vi "SaveRawData.vi"(4 "error in (no error)":errorcluster, 6 "raw data to be saved":T1[](array[typedef]), 7 "path in":path) -> (0 "error out":errorcluster, 3 "path out":path)   [LabVIEW 2020, in "Initialization.lvlib" / "FileManagement.lvlib"]
uses:
  FileManagement.lvlib
  SignalConversion/DAQChannelRawData.ctl
  SignalConversion/SignalConverson.lvlib
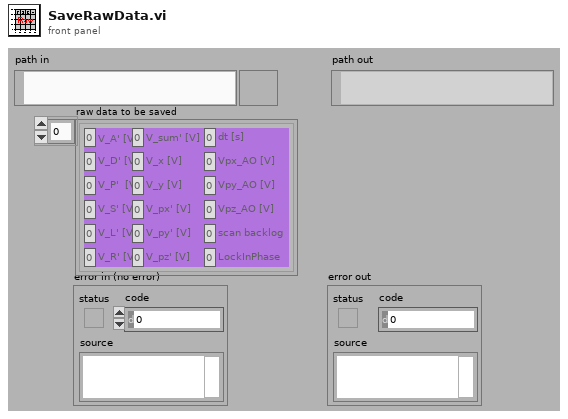
[diagram p1: front panel]
types:
  T1 = typedef "SignalConverson.lvlib/DAQChannelRawData.ctl" = cluster{"V_A' [V]":dbl, "V_D' [V]":dbl, "V_P'  [V]":dbl, "V_S' [V]":dbl, "V_L' [V]":dbl, "V_R' [V]":dbl, "V_sum' [V]":dbl, "V_x [V]":dbl, "V_y [V]":dbl, "V_px' [V]":dbl, "V_py' [V]":dbl, "V_pz' [V]":dbl, "dt [s]":dbl, "Vpx_AO [V]":dbl, "Vpy_AO [V]":dbl, "Vpz_AO [V]":dbl, "scan backlog":u32, "LockInPhase":dbl}
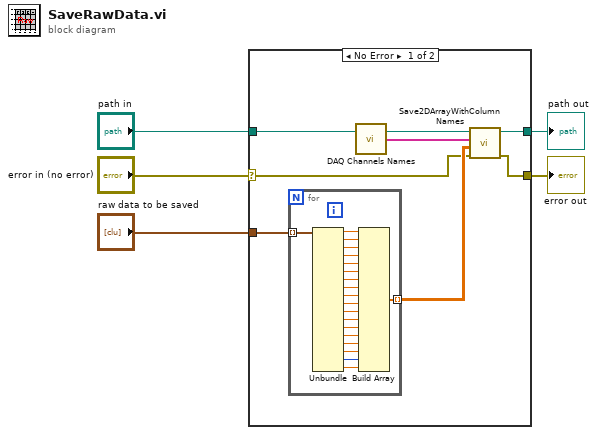
[diagram p0: block diagram]
diagram:
  n1 = case shown="No Error" "error in (no error)" {
    selector: "error in (no error)" -> [w10 w34]
    tunnel: "path in" -> [w8 w33]
    tunnel: "raw data to be saved" -> [w12 _]
    tunnel: [w6 w33] -> w4
    tunnel: [w7 w34] -> w3
    frame No Error {
      n2 = for {
        tunnel: w12 -> [w32] mode=indexing
        tunnel: [w13] -> w11 mode=indexing
        n3 = Unbundle(w32) -> ("V_A' [V]"=w31:dbl, "V_D' [V]"=w30:dbl, "V_P'  [V]"=w29:dbl, "V_S' [V]"=w28:dbl, "V_L' [V]"=w27:dbl, "V_R' [V]"=w26:dbl, "V_sum' [V]"=w25:dbl, "V_x [V]"=w24:dbl, "V_y [V]"=w23:dbl, "V_px' [V]"=w22:dbl, "V_py' [V]"=w21:dbl, "V_pz' [V]"=w20:dbl, "dt [s]"=w19:dbl, "Vpx_AO [V]"=w18:dbl, "Vpy_AO [V]"=w17:dbl, "Vpz_AO [V]"=w16:dbl, "scan backlog"=w15:u32, "LockInPhase"=w14:dbl)
        n4 = Build Array(w31, w30, w29, w28, w27, w26, w25, w24, w23, w22, w21, w20, w19, w18, w17, w16, w15, w14) -> (w13:dbl[])
      }
      n5 = call "DAQ Channels Names.vi"() -> ("DAQ channel names (string)"=w9:string[])  [unwired: 7 in]
      n6 = call "Save2DArrayWithColumnNames.vi"("error in (no error)"=w10, "2D data"=w11, "Column name array"=w9, "path in"=w8) -> ("error out"=w7:errorcluster, "path out"=w6:path)  [unwired: 6 in]
    }
    frame Error {
    }
  }
  "path out" <- w4
  "error out" <- w3
